vi "Retry RUN.vi"(8 "error in (no error)":errorcluster, 10 "Next?":bool=TRUE, 11 "Monkey in":refnum<class "Monkey.lvclass">) -> (0 "error out":errorcluster, 3 "Monkey out":refnum<class "Monkey.lvclass">)   [LabVIEW 2020, in "TALOS.lvlib" / "Monkey.lvlib" / "Monkey.lvclass"]
doc: "Retry the last script"
uses:
  Monkey.lvclass
  Run Utilities/Run Block/Run Block.lvclass
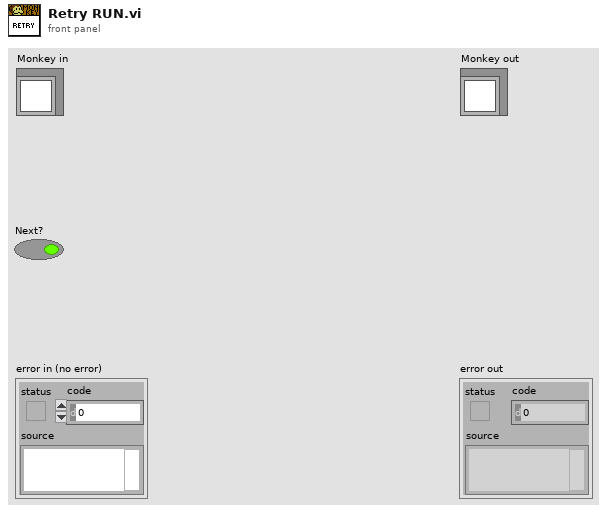
[diagram p1: front panel]
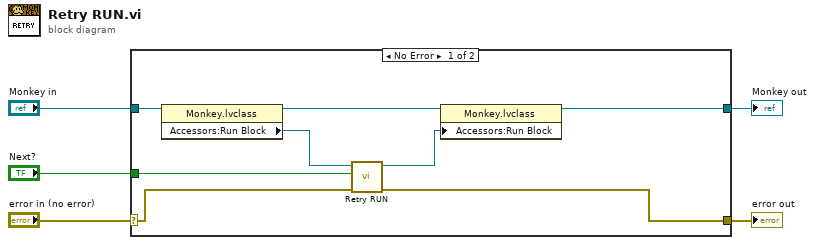
[diagram p0: block diagram]
diagram:
  n1 = case shown="No Error" "error in (no error)" {
    selector: "error in (no error)" -> [w8 w15]
    tunnel: [w7 w15] -> w4
    tunnel: [w10 w14] -> w2
    tunnel: "Monkey in" -> [w13 w14]
    tunnel: "Next?" -> [w6 _]
    frame No Error {
      n2 = property class="Monkey.lvclass"(reference=w13) -> (reference out=w12:refnum<class "Monkey.lvclass">, "Accessors:Run Block"=w11:refnum<class "Run Block.lvclass">)  [unwired: 1 in, 1 out]
      n3 = call-dynamic "Retry RUN.vi"("error in (no error)"=w8, "Next?"=w6, "Run Block in"=w11) -> ("error out"=w7:errorcluster, "Run Block out"=w9:refnum<class "Run Block.lvclass">)  [unwired: 7 in]
      n4 = property class="Monkey.lvclass"(reference=w12, "Accessors:Run Block"=w9) -> (reference out=w10:refnum<class "Monkey.lvclass">)  [unwired: 1 in, 1 out]
    }
    frame Error {
    }
  }
  "error out" <- w4
  "Monkey out" <- w2
